vi "Motion Virtual Front Panel_libESP301.vi"() -> ()   [LabVIEW 2015, in "Newport ESP301.lvlib"]
doc: "Motion Virtual Front Panel:\n\nThis is a sample of an application that can be built with the LabVIEW drivers.\n\nPress HOME / ENABLE in top left of panel to put stage in Ready state for motion."
uses:
  <userlib>/Newport ESP301/Newport ESP301.lvlib
  <vilib>/Platform/TimedLoop/XDataNode/timing_clust.ctl
  <vilib>/Platform/TimedLoop/XDataNode/nitl_modes.ctl
  <vilib>/Platform/TimedLoop/XDataNode/wakeup.ctl
  <vilib>/Platform/TimedLoop/XDataNode/XDataNode.xnode
  <vilib>/Platform/TimedLoop/XDataNode/XDNodeRunTimeDep.lvlib
panel:
  out "Title":string
  out "counter":i32
  in  "Set Max":bool
  in  "Set Min":bool
  in  "Max":dbl
  in  "Min":dbl
  in  "Set velocity":bool
  out "Stop cycle":bool=TRUE
  out "Title 2":string
  in  "Cycle":bool
  in  "# Loops":i32=5
  in  "Go2":bool
  in  "Go1":bool
  in  "Abs. Move 2":dbl=1.0
  in  "Abs. Move 1":dbl
  in  "-":bool
  in  "+":bool
  in  "Step":dbl
  out "Position History":dbl(graph)=1.5
  in  "Action":bool
  out "Stop polling":bool=TRUE
  out "Controller state description":string="STATUS"
  out "Velocity MAX":dbl=0.4
  out "Controller state":string="33"
  out "Positioner error":string="0000"
  in  "Velocity:":dbl
  in  "Exit":bool=TRUE
  out "Target position":dbl
  in  "Position glissière":cluster{dbl, dbl}(slide) scale=-45.0..45.0
  in  "Exit":bool
  out "Current position":dbl
  # "unit/s"
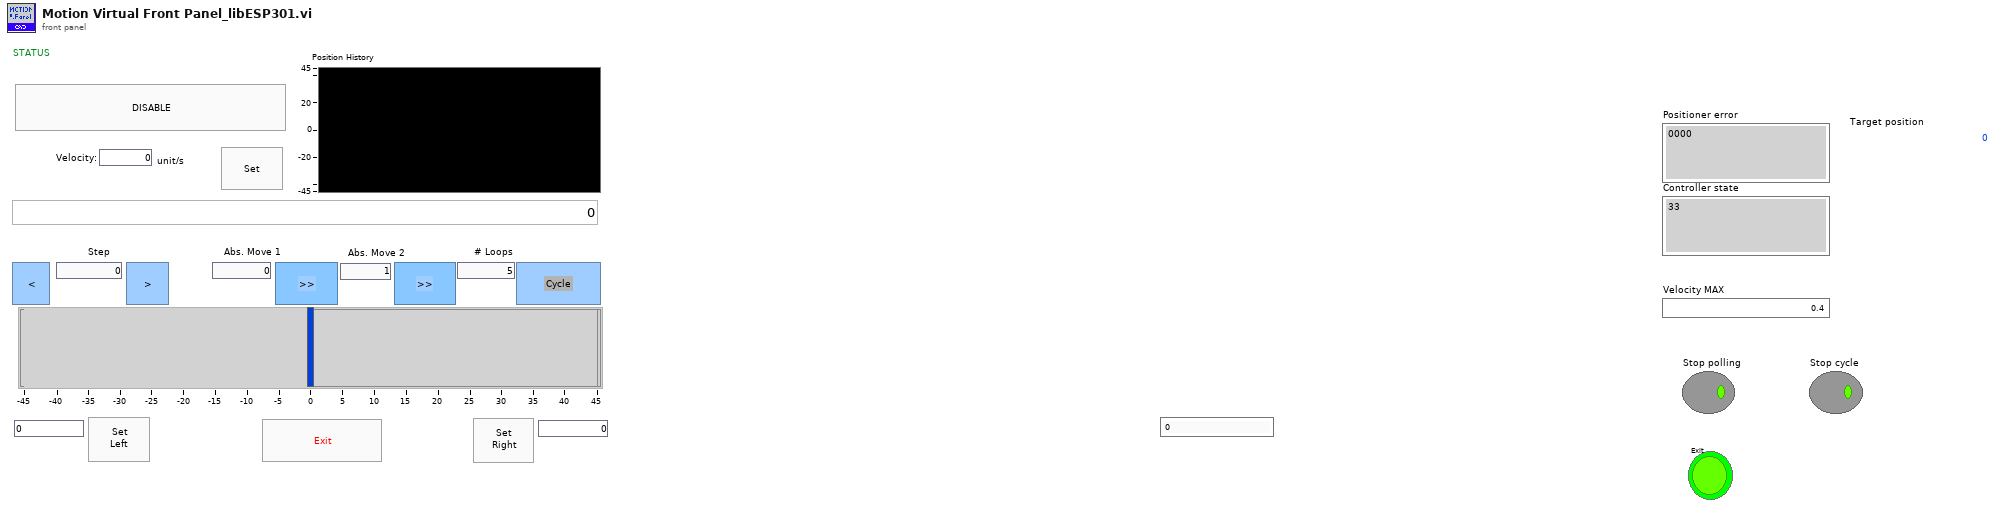
[diagram p1: front panel]
types:
  T1 = typedef "XDNodeRunTimeDep.lvlib/timing_clust.ctl" = cluster{"Expected End [f-1]":u64, "Actual End [f-1]":u64, "Finished Late? [f-1]":bool, "Expected End [i-1]":u64, "Actual End [i-1]":u64, "Finished Late? [i-1]":bool, "Expected Start [i]":u64, "Actual Start [i]":u64, "Expected Start [f]":u64, "Actual Start [f]":u64, "Source Name":string, "Structure Name":string, "Period":i64, "Deadline":i64, "Offset":i64, "Start":i64, "Priority":i32, "Timeout":i32, "Mode":T2, "Wakeup Reason":T3, "Error":errorcluster, "Source Type":string, "Secondary Source Type":string, "Global End Time":u64, "Global Start Time":u64, "Frame Duration":u64, "Iteration Duration":u64, "Assigned CPU":i32, "I/O Scan Engine Mode":u32}
  T2 = typedef "XDNodeRunTimeDep.lvlib/nitl_modes.ctl" = enum32{"No Change", "Process missed periods, maintain original phase", "Discard missed periods, maintain original phase", "Process missed periods, ignore original phase", "Discard missed periods, ignore original phase"}
  T3 = typedef "XDNodeRunTimeDep.lvlib/wakeup.ctl" = enum32{"Normal", "Aborted", "Asynchronous wakeup", "Timing source error", "Timed loop error", "Timeout"}
  T4 = cluster{"VISA resource name":refnum<visa-resource-name>, "Device name":string, "Controller address":i32, "error":errorcluster}
  T5 = cluster{"Axis1 moving":bool, "Axis2 moving":bool, "Axis3 moving":bool, "Axis4 moving":bool, "Motor Power of at least one axis":bool, "Reserved":bool, "Reserved":bool, "Reserved":bool, "Axis5 moving 2":bool, "Axis6 moving 2":bool, "Reserved":bool, "Reserved":bool, "Motor Power of at least one axis":bool, "Reserved":bool, "Reserved":bool, "Reserved":bool}
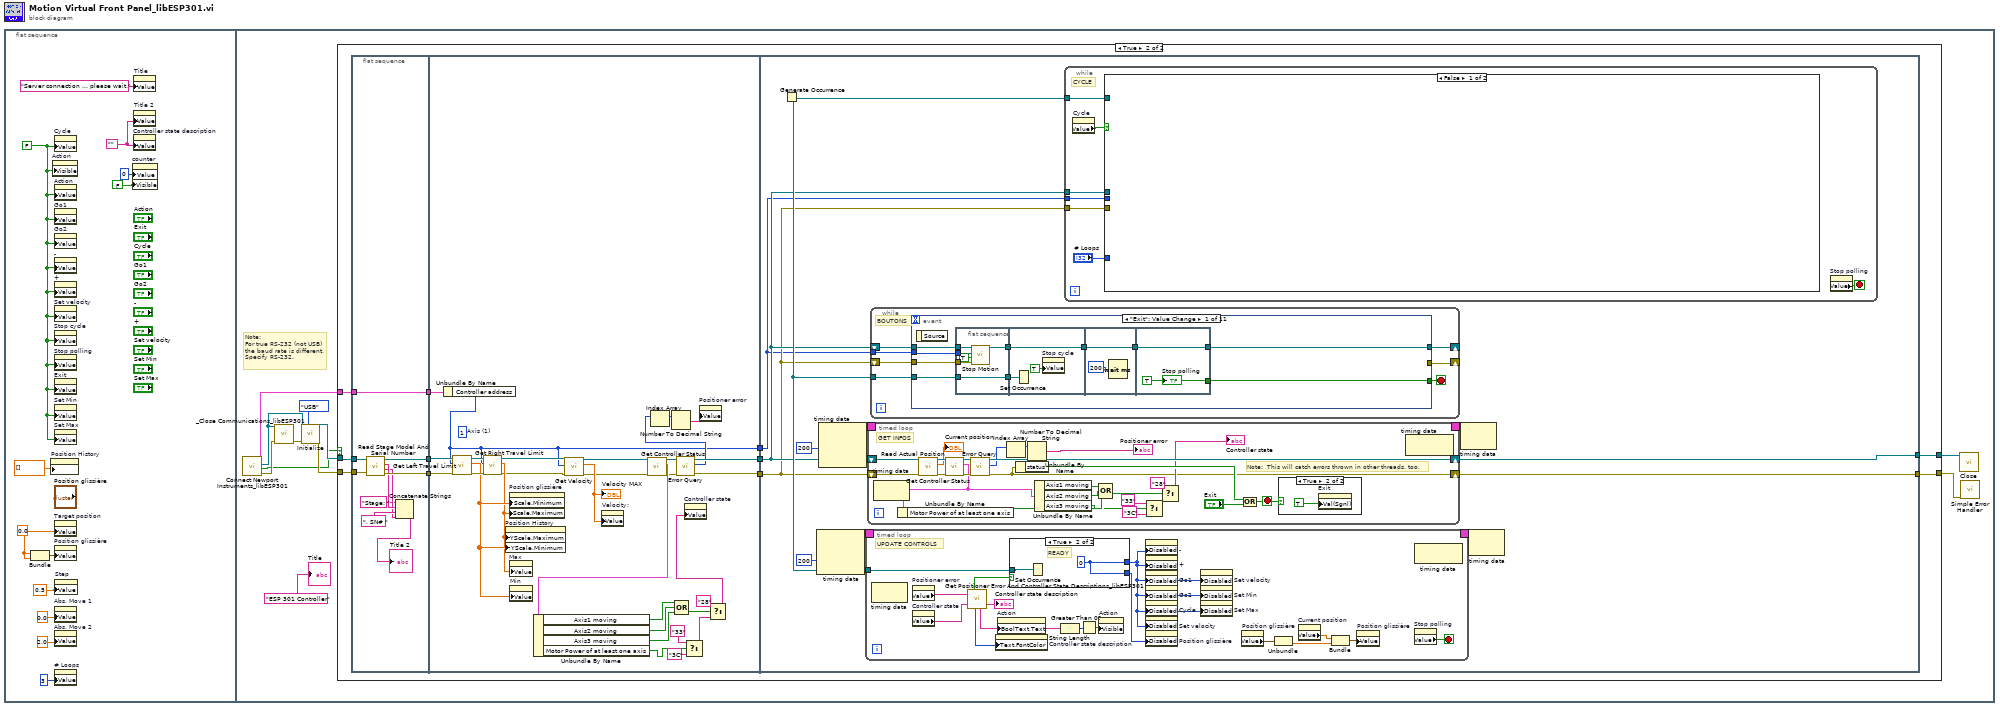
[diagram p0: block diagram]
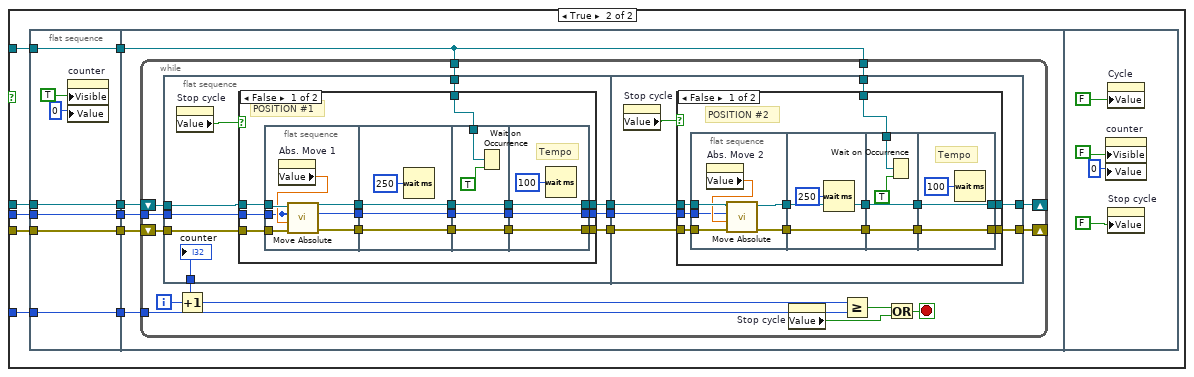
[diagram p3: hidden frame]
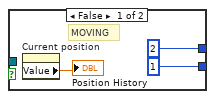
[diagram p6: hidden frame]
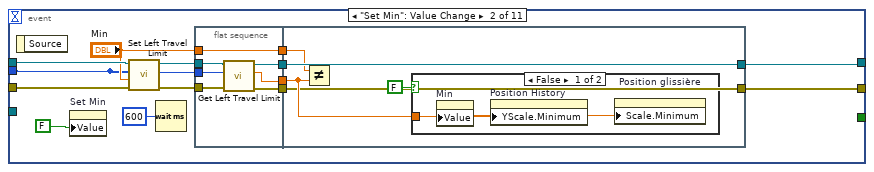
[diagram p7: hidden frame]
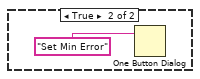
[diagram p8: hidden frame]
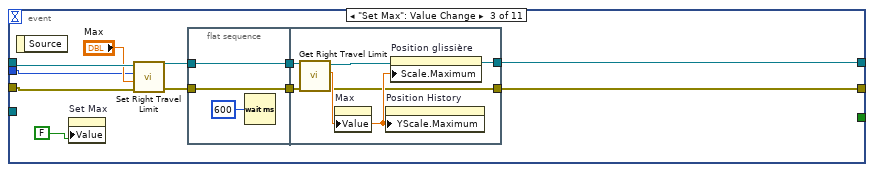
[diagram p9: hidden frame]
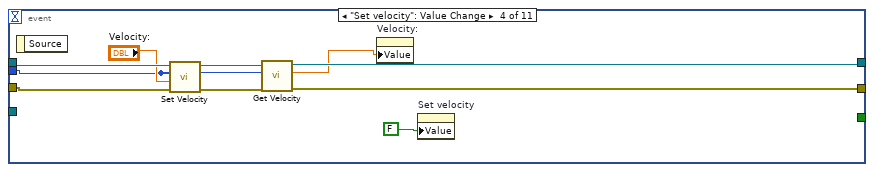
[diagram p10: hidden frame]
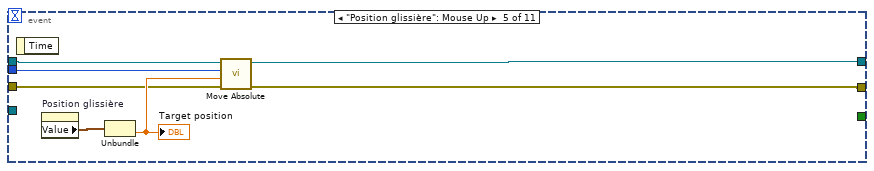
[diagram p11: hidden frame]
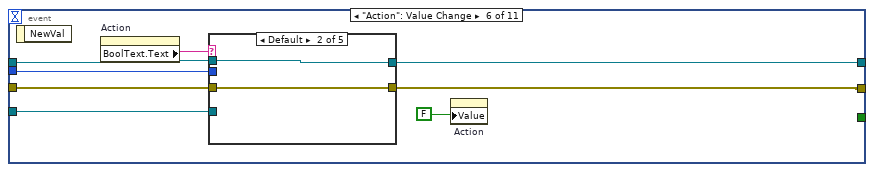
[diagram p12: hidden frame]
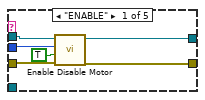
[diagram p13: hidden frame]
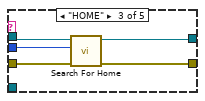
[diagram p14: hidden frame]
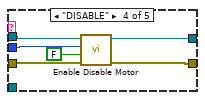
[diagram p15: hidden frame]
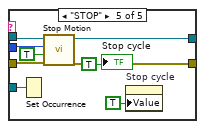
[diagram p16: hidden frame]
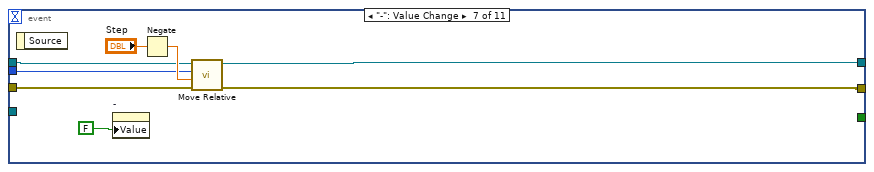
[diagram p17: hidden frame]
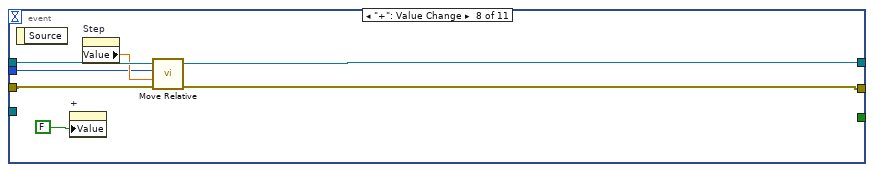
[diagram p18: hidden frame]
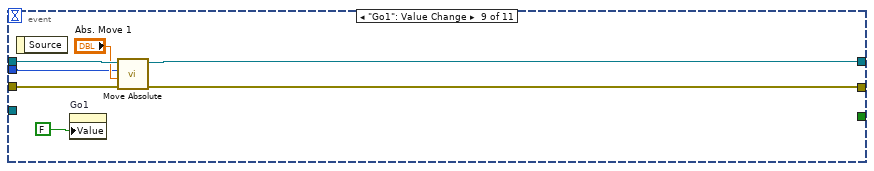
[diagram p19: hidden frame]
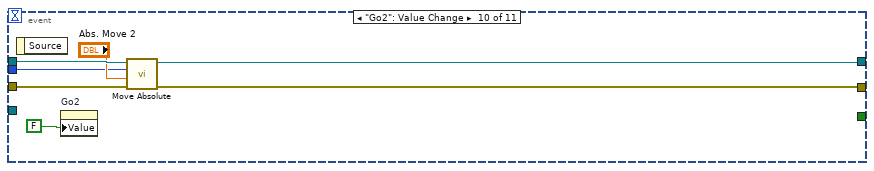
[diagram p20: hidden frame]
diagram:
  n1 = flat-sequence {
    frame #0 {
      w8 = FALSE
      w11 = 0.0
      w10 = ""
      n2 = Bundle(w11, w11) -> (w12:cluster{dbl, dbl})  [unwired: 1 out]
      n3 = property on="Position History" class="WFChart (strict)"("History Data"=dbl[] [] ("Données d'historique")) -> ()  [unwired: 2 in, 2 out]
      n4 = property on="Action" class="Bool (strict)"("Visible"=w8) -> ()  [unwired: 2 in, 2 out]
      n5 = property on="Cycle" class="Bool (strict)"("Value"=w8) -> ()  [unwired: 2 in, 2 out]
      n6 = property on="Action" class="Bool (strict)"("Value"=w8) -> ()  [unwired: 2 in, 2 out]
      n7 = property on="Go1" class="Bool (strict)"("Value"=w8) -> ()  [unwired: 2 in, 2 out]
      n8 = property on="Go2" class="Bool (strict)"("Value"=w8) -> ()  [unwired: 2 in, 2 out]
      n9 = property on="-" class="Bool (strict)"("Value"=w8) -> ()  [unwired: 2 in, 2 out]
      n10 = property on="+" class="Bool (strict)"("Value"=w8) -> ()  [unwired: 2 in, 2 out]
      n11 = property on="Set velocity" class="Bool (strict)"("Value"=w8) -> ()  [unwired: 2 in, 2 out]
      n12 = property on="Stop cycle" class="Bool (strict)"("Value"=w8) -> ()  [unwired: 2 in, 2 out]
      n13 = property on="Stop polling" class="Bool (strict)"("Value"=w8) -> ()  [unwired: 2 in, 2 out]
      n14 = property on="Exit" class="Bool (strict)"("Value"=w8) -> ()  [unwired: 2 in, 2 out]
      n15 = property on="Set Min" class="Bool (strict)"("Value"=w8) -> ()  [unwired: 2 in, 2 out]
      n16 = property on="Set Max" class="Bool (strict)"("Value"=w8) -> ()  [unwired: 2 in, 2 out]
      n17 = property on="Target position" class="DigNum (strict)"("Value"=w11) -> ()  [unwired: 2 in, 2 out]
      n18 = property on="Position glissière" class="Slide (strict)"("Value"=w12) -> ()  [unwired: 2 in, 2 out]
      n19 = property on="Abs. Move 1" class="DigNum (strict)"("Value"=0.0 ("Abs. Move 1")) -> ()  [unwired: 2 in, 2 out]
      n20 = property on="Abs. Move 2" class="DigNum (strict)"("Value"=2.0 ("Abs. Move 2")) -> ()  [unwired: 2 in, 2 out]
      n21 = property on="# Loops" class="DigNum (strict)"("Value"=3 ("# Loops")) -> ()  [unwired: 2 in, 2 out]
      n22 = property on="Step" class="DigNum (strict)"("Value"=0.5 ("Step")) -> ()  [unwired: 2 in, 2 out]
      n23 = property on="counter" class="DigNum (strict)"("Value"=0 ("counter"), "Visible"=FALSE) -> ()  [unwired: 2 in, 2 out]
      n24 = property on="Title" class="Str"("Value"="Server connection ... please wait." ("Title")) -> ()  [unwired: 2 in, 2 out]
      n25 = property on="Title 2" class="Str"("Value"=w10) -> ()  [unwired: 2 in, 2 out]
      n26 = property on="Controller state description" class="Str"("Value"=w10) -> ()  [unwired: 2 in, 2 out]
    }
    frame #1 {
      # "Note:\nFor true RS-232 (not USB)\nthe baud rate is different.\nSpecify RS-232."
      n27 = call <userlib>:"Connect Newport Instruments_libESP301.vi"() -> ("error (duplicate)"=w16:errorcluster, "Connected"=w15:bool, "VISA resource name (duplicate)"=w14:refnum<visa-resource-name>, "Device Connection Cluster"=w13:T4)  [unwired: 7 in, 1 out]
      n28 = call <userlib>:"_Close Communications_libESP301.vi"("Instrument Channel"=w14, "error in (no error)"=w16) -> ("error out"=w22:errorcluster)  [unwired: 13 in]
      n29 = call <userlib>:"Initialize.vi"("VISA resource name"=w14, "error in (no error)"=w22, "Serial Link (USB)"=enum16{"RS232", "USB"}."USB" ("Serial Link (RS232)")) -> ("VISA resource name out"=w20:refnum<visa-resource-name>, "error out"=w19:errorcluster)  [unwired: 6 in]
      n30 = case shown="True" w15 {
        tunnel: w20 -> [w25 w35]
        tunnel: [w25 w33] -> w23
        tunnel: w19 -> [w24 w32]
        tunnel: [w24 w28] -> w18
        tunnel: w13 -> [_ w27]
        frame False {
        }
        frame True {
          n31 = flat-sequence {
            tunnel: w35 -> [w46]
            tunnel: [w45] -> w34
            tunnel: w32 -> [w44]
            tunnel: [w43] -> w31
            tunnel: w27 -> [w37]
            tunnel: [w37] -> w26
            tunnel: [w66] -> w36
            tunnel: w34 -> [w77]
            tunnel: w31 -> [w75]
            tunnel: [w49] -> w30
            tunnel: [w47] -> w29
            tunnel: w26 -> [w48]
            tunnel: [w89] -> w33
            tunnel: [w88] -> w28
            tunnel: w29 -> [w78]
            tunnel: w30 -> [w79]
            tunnel: w36 -> [w80]
            frame #0 {
              n32 = call <userlib>:"Read Stage Model And Serial Number.vi"("error in (no error)"=w44, "VISA resource name"=w46) -> ("error out"=w43:errorcluster, "Serial number"=w40:string, "Model number"=w41:string, "VISA resource name out"=w45:refnum<visa-resource-name>)  [unwired: 2 in]
              n33 = Concatenate Strings("Stage: " ("string"), w41, ", SN# " ("string"), w40) -> (→"Title 2":string)
            }
            frame #1 {
              (unwired) 1  # Axis (1)
              n34 = Unbundle By Name(w48) -> ("Controller address"=w47:i32)
              n35 = call <userlib>:"Get Left Travel Limit.vi"("error in (no error)"=w75, "Axis (1)"=w47, "VISA resource name"=w77) -> ("error out"=w74:errorcluster, "Left Travel Limit (units)"=w73:dbl, "VISA resource name out"=w76:refnum<visa-resource-name>)  [unwired: 2 in]
              n36 = call <userlib>:"Get Right Travel Limit.vi"("error in (no error)"=w74, "Axis (1)"=w47, "VISA resource name"=w76) -> ("error out"=w68:errorcluster, "Right Travel Limit (units)"=w72:dbl, "VISA resource name out"=w71:refnum<visa-resource-name>)  [unwired: 2 in]
              n37 = property on="Position History" class="WFChart (strict)"("YScale.Maximum"=w72, "YScale.Minimum"=w73) -> ()  [unwired: 2 in, 2 out]
              n38 = property on="Position glissière" class="Slide (strict)"("Scale.Minimum"=w73, "Scale.Maximum"=w72) -> ()  [unwired: 2 in, 2 out]
              n39 = property on="Max" class="DigNum (strict)"("Value"=w72) -> ()  [unwired: 2 in, 2 out]
              n40 = property on="Min" class="DigNum (strict)"("Value"=w73) -> ()  [unwired: 2 in, 2 out]
              n41 = call <userlib>:"Get Velocity.vi"("error in (no error)"=w68, "Axis (1)"=w47, "VISA resource name"=w71) -> ("error out"=w51:errorcluster, "Velocity (units/s)"=w69:dbl, "VISA resource name out"=w70:refnum<visa-resource-name>)  [unwired: 2 in]
              "Velocity MAX" <- w69
              n42 = property on="Velocity:" class="DigNum (strict)"("Value"=w69) -> ()  [unwired: 2 in, 2 out]
              n43 = call <userlib>:"Get Controller Status.vi"("error in (no error)"=w51, "VISA resource name"=w70) -> ("error out"=w50:errorcluster, "Controller Status"=w62:T5, "VISA resource name out"=w67:refnum<visa-resource-name>)  [unwired: 2 in, 1 out]
              n44 = Unbundle By Name(w62) -> ("Axis1 moving"=w61:bool, "Axis2 moving"=w60:bool, "Axis3 moving"=w59:bool, "Motor Power of at least one axis"=w52:bool)
              n45 = Compound Arithmetic op=OR(w61, w60, w59) -> (w58:bool)
              n46 = call <userlib>:"Error Query.vi"("error in (no error)"=w50, "VISA resource name"=w67) -> ("error out"=w49:errorcluster, "Error Code"=w64:i32[], "VISA resource name out"=w66:refnum<visa-resource-name>)  [unwired: 2 in, 1 out]
              n47 = Index Array(array=w64) -> (element=w65:i32)  [unwired: 1 in]
              n48 = Number To Decimal String(number=w65) -> (decimal integer string=w63:string)  [unwired: 1 in]
              n49 = Select(t="33" ("f"), s=w52, f="3C") -> (s? t:f=w54:string)
              n50 = property on="Positioner error" class="Str"("Value"=w63) -> ()  [unwired: 2 in, 2 out]
              n51 = Select(t="28", s=w58, f=w54) -> (s? t:f=w56:string)
              n52 = property on="Controller state" class="Str"("Value"=w56) -> ()  [unwired: 2 in, 2 out]
            }
            frame #2 {
              n53 = Generate Occurrence() -> (w81:refnum<k4>)
              n54 = node-c288(i64 200 ("Période")) -> (w85:T1)  [unwired: 1 in, 1 out]
              n55 = node-c288(i64 200 ("Période")) -> (w87:T1)  [unwired: 1 in, 1 out]
              n56 = timed-loop {
                timing: w85 -> [_]
                timing-out: [_] -> w84
                tunnel: w81 -> [w227]
                stop <- w229 stop-if-true
                # "UPDATE CONTROLS"
                n57 = node-c288() -> ()  [unwired: 2 out]
                n58 = property on="Positioner error" class="Str"() -> ("Value"=w238:string)  [unwired: 2 in, 2 out]
                n59 = property on="Controller state" class="Str"() -> ("Value"=w237:string)  [unwired: 2 in, 2 out]
                n60 = call <userlib>:"Get Positioner Error And Controller State Descriptions_libESP301.vi"("Controller state"=w237, "Positioner error"=w238) -> ("Color"=w235:u32, "Action name"=w234:string, "Controller state description"=→"Controller state description":string, "IsReady?"=w231:bool)  [unwired: 2 out]
                n61 = property on="Controller state description" class="Str"("Text.FontColor"=w235) -> ()  [unwired: 2 in, 2 out]
                n62 = property on="Action" class="Bool (strict)"("BoolText.Text"=w234) -> ()  [unwired: 2 in, 2 out]
                n63 = case shown="True" w231 {
                  tunnel: [u8 2 w243] -> w228
                  tunnel: [u8 1 w243] -> w230
                  tunnel: w227 -> [_ w242]
                  frame False {
                    # "MOVING"
                    n64 = property on="Current position" class="DigNum (strict)"() -> ("Value"=→"Position History":dbl)  [unwired: 2 in, 2 out]
                  }
                  frame True {
                    w243 = u8 0
                    # "READY"
                    n65 = Set Occurrence(w242) -> ()
                  }
                }
                n66 = String Length(string=w234) -> (length=w233:i32)
                n67 = Greater Than 0?(x=w233) -> (x > 0?=w232:bool)
                n68 = property on="Action" class="Bool (strict)"("Visible"=w232) -> ()  [unwired: 2 in, 2 out]
                n69 = property on="-" class="Bool (strict)"("Disabled"=w228) -> ()  [unwired: 2 in, 2 out]
                n70 = property on="+" class="Bool (strict)"("Disabled"=w228) -> ()  [unwired: 2 in, 2 out]
                n71 = property on="Go1" class="Bool (strict)"("Disabled"=w228) -> ()  [unwired: 2 in, 2 out]
                n72 = property on="Go2" class="Bool (strict)"("Disabled"=w228) -> ()  [unwired: 2 in, 2 out]
                n73 = property on="Cycle" class="Bool (strict)"("Disabled"=w228) -> ()  [unwired: 2 in, 2 out]
                n74 = property on="Set velocity" class="Bool (strict)"("Disabled"=w228) -> ()  [unwired: 2 in, 2 out]
                n75 = property on="Position glissière" class="Slide (strict)"("Disabled"=w230) -> ()  [unwired: 2 in, 2 out]
                n76 = property on="Set velocity" class="Bool (strict)"("Disabled"=w228) -> ()  [unwired: 2 in, 2 out]
                n77 = property on="Set Min" class="Bool (strict)"("Disabled"=w228) -> ()  [unwired: 2 in, 2 out]
                n78 = property on="Set Max" class="Bool (strict)"("Disabled"=w228) -> ()  [unwired: 2 in, 2 out]
                n79 = property on="Position glissière" class="Slide (strict)"() -> ("Value"=w224:cluster{dbl, dbl})  [unwired: 2 in, 2 out]
                n80 = Unbundle(w224) -> (w223:dbl)  [unwired: 1 out]
                n81 = property on="Current position" class="DigNum (strict)"() -> ("Value"=w225:dbl)  [unwired: 2 in, 2 out]
                n82 = Bundle("Value"=w225, w223) -> (w226:cluster{"Value":dbl, dbl})  [unwired: 1 out]
                n83 = property on="Position glissière" class="Slide (strict)"("Value"=w226) -> ()  [unwired: 2 in, 2 out]
                n84 = node-c288() -> ()  [unwired: 2 out]
                n85 = property on="Stop polling" class="Bool (strict)"() -> ("Value"=w229:bool)  [unwired: 2 in, 2 out]
              }
              n86 = timed-loop {
                timing: w87 -> [_]
                timing-out: [_] -> w86
                shift-right: [w427] -> w89
                shift-left: w80 -> [w434]
                shift-right: [w411] -> w88
                shift-left: w79 -> [w412]
                stop <- w436 stop-if-true
                # "Note:  This will catch errors thrown in other threads, too."
                # "GET INFOS"
                n87 = node-c288() -> ()  [unwired: 2 out]
                n88 = call <userlib>:"Read Actual Position.vi"("error in (no error)"=w412, "VISA resource name"=w434) -> ("error out"=w431:errorcluster, "Position (units)"=→"Current position":dbl, "VISA resource name out"=w433:refnum<visa-resource-name>)  [unwired: 3 in]
                n89 = call <userlib>:"Get Controller Status.vi"("error in (no error)"=w431, "VISA resource name"=w433) -> ("error out"=w428:errorcluster, "Controller Status"=w417:T5, "VISA resource name out"=w429:refnum<visa-resource-name>)  [unwired: 2 in, 1 out]
                n90 = Unbundle By Name(w417) -> ("Motor Power of at least one axis"=w416:bool)
                n91 = call <userlib>:"Error Query.vi"("error in (no error)"=w428, "VISA resource name"=w429) -> ("error out"=w411:errorcluster, "Error Code"=w426:i32[], "VISA resource name out"=w427:refnum<visa-resource-name>)  [unwired: 2 in, 1 out]
                n92 = Index Array(array=w426) -> (element=w425:i32)  [unwired: 1 in]
                n93 = Unbundle By Name(w411) -> ("status"=w430:bool)
                n94 = Number To Decimal String(number=w425) -> (decimal integer string=→"Positioner error":string)  [unwired: 1 in]
                n95 = Unbundle By Name(w417) -> ("Axis1 moving"=w419:bool, "Axis2 moving"=w420:bool, "Axis3 moving"=w421:bool)
                n96 = Compound Arithmetic op=OR(w419, w420, w421) -> (w422:bool)
                n97 = Select(t="33" ("f"), s=w416, f="3C") -> (s? t:f=w413:string)
                n98 = Select(t="28", s=w422, f=w413) -> (s? t:f=→"Controller state":string)
                n99 = Or(x=w430, y="Exit") -> (x .or. y?=w436:bool)
                n100 = case shown="True" w436 {
                  frame False {
                  }
                  frame True {
                    n101 = property on="Exit" class="Bool (strict)"("Val(Sgnl)"=TRUE) -> ()  [unwired: 2 in, 2 out]
                  }
                }
                n102 = node-c288() -> ()  [unwired: 2 out]
              }
              n103 = while {
                shift-right: [w256] -> _
                shift-left: w80 -> [w255]
                tunnel: w81 -> [w253]
                tunnel: w78 -> [w251]
                shift-right: [w250] -> _
                shift-left: w79 -> [w252]
                stop <- w254 stop-if-true
                # "BOUTONS"
                n104 = event shown="[0] \"Exit\": Value Change" {
                  selector: _ -> [_ _ _ _ _ _ _ _ _ _ _]
                  dyn-events: _ -> [_ _ _ _ _ _ _ _ _ _ _]
                  timeout: _ -> [_ _ _ _ _ _ _ _ _ _ _]
                  tunnel: [w264 _ _ _ _ _ _ _ _ _ _] -> w254
                  tunnel: w255 -> [w259 w287 w315 w335 w342 w350 w384 w392 w400 w406 w409]
                  tunnel: [w266 w292 w316 w333 w341 w349 w383 w393 w399 w407 w409] -> w256
                  tunnel: w253 -> [w261 _ _ _ _ w347 _ _ _ _ _]
                  tunnel: w252 -> [w257 w283 w312 w330 w338 w346 w382 w390 w397 w404 _]
                  tunnel: w251 -> [w258 w284 w311 w327 w339 w345 w381 w389 w395 w403 _]
                  tunnel: [_ w281 w308 w328 w337 w344 w380 w388 w396 w402 _] -> w250
                  event "Exit": Value Change {
                    n105 = event-data() -> ()  [unwired: 2 out]
                    n106 = flat-sequence {
                      tunnel: [w270] -> w265
                      tunnel: w261 -> [w272]
                      tunnel: [w272] -> w260
                      tunnel: w259 -> [w271]
                      tunnel: w258 -> [w268]
                      tunnel: w257 -> [w267]
                      tunnel: w265 -> [w275]
                      tunnel: [w275] -> w263
                      tunnel: w260 -> [w273]
                      tunnel: w263 -> [w277]
                      tunnel: [w277] -> w262
                      tunnel: [w279] -> w266
                      tunnel: w262 -> [w279]
                      tunnel: [w278] -> w264
                      frame #0 {
                        n107 = call <userlib>:"Stop Motion.vi"("error in (no error)"=w267, "Stop all axes (F)"=TRUE, "Axis (1)"=w268, "VISA resource name"=w271) -> ("VISA resource name out"=w270:refnum<visa-resource-name>)  [unwired: 2 in, 1 out]
                      }
                      frame #1 {
                        n108 = Set Occurrence(w273) -> ()
                        n109 = property on="Stop cycle" class="Bool (strict)"("Value"=TRUE) -> ()  [unwired: 2 in, 2 out]
                      }
                      frame #2 {
                        n110 = Wait (ms)(milliseconds to wait=u32 200 ("attente (ms)")) -> ()  [unwired: 1 out]
                      }
                      frame #3 {
                        w278 = TRUE
                        "Stop polling" <- w278
                      }
                    }
                  }
                  event "Set Min": Value Change {
                    n111 = event-data() -> ()  [unwired: 2 out]
                    n112 = property on="Set Min" class="Bool (strict)"("Value"=FALSE ("Set Min")) -> ()  [unwired: 2 in, 2 out]
                    n113 = call <userlib>:"Set Left Travel Limit.vi"("error in (no error)"=w283, "Left Travel Limit"="Min", "Axis (1)"=w284, "VISA resource name"=w287) -> ("error out"=w282:errorcluster, "VISA resource name out"=w286:refnum<visa-resource-name>)  [unwired: 2 in]
                    n114 = Wait (ms)(milliseconds to wait=u32 600 ("attente (ms)")) -> ()  [unwired: 1 out]
                    n115 = flat-sequence {
                      tunnel: [w298] -> w290
                      tunnel: [w300] -> w289
                      tunnel: "Min" -> [w300]
                      tunnel: [w297] -> w288
                      tunnel: w286 -> [w299]
                      tunnel: w284 -> [w296]
                      tunnel: w282 -> [w295]
                      tunnel: [w294] -> w280
                      tunnel: [w305] -> w292
                      tunnel: w290 -> [w305]
                      tunnel: w289 -> [w304]
                      tunnel: w288 -> [w302]
                      tunnel: [w301] -> w281
                      tunnel: w280 -> [w301]
                      frame #0 {
                        n116 = call <userlib>:"Get Left Travel Limit.vi"("error in (no error)"=w295, "Axis (1)"=w296, "VISA resource name"=w299) -> ("error out"=w294:errorcluster, "Left Travel Limit (units)"=w297:dbl, "VISA resource name out"=w298:refnum<visa-resource-name>)  [unwired: 2 in]
                      }
                      frame #1 {
                        n117 = Not Equal?(x=w304, y=w302) -> ()  [unwired: 1 out]
                        n118 = case shown="False" FALSE {
                          tunnel: w302 -> [w306 _]
                          frame False {
                            n119 = property on="Min" class="DigNum (strict)"("Value"=w306) -> ()  [unwired: 2 in, 2 out]
                            n120 = property on="Position History" class="WFChart (strict)"("YScale.Minimum"=w306) -> ()  [unwired: 2 in, 2 out]
                            n121 = property on="Position glissière" class="Slide (strict)"("Scale.Minimum"=w306) -> ()  [unwired: 2 in, 2 out]
                          }
                          frame True {
                            n122 = One Button Dialog(message="Set Min Error") -> ()  [unwired: 1 in, 1 out]
                          }
                        }
                      }
                    }
                  }
                  event "Set Max": Value Change {
                    n123 = event-data() -> ()  [unwired: 2 out]
                    n124 = property on="Set Max" class="Bool (strict)"("Value"=FALSE ("Set Max")) -> ()  [unwired: 2 in, 2 out]
                    n125 = call <userlib>:"Set Right Travel Limit.vi"("error in (no error)"=w312, "Right Travel Limit"="Max", "Axis (1)"=w311, "VISA resource name"=w315) -> ("error out"=w310:errorcluster, "VISA resource name out"=w314:refnum<visa-resource-name>)  [unwired: 2 in]
                    n126 = flat-sequence {
                      tunnel: w314 -> [w321]
                      tunnel: [w321] -> w317
                      tunnel: w310 -> [w319]
                      tunnel: [w319] -> w309
                      tunnel: [w325] -> w316
                      tunnel: w317 -> [w326]
                      tunnel: w309 -> [w323]
                      tunnel: [w322] -> w308
                      frame #0 {
                        n127 = Wait (ms)(milliseconds to wait=u32 600 ("attente (ms)")) -> ()  [unwired: 1 out]
                      }
                      frame #1 {
                        n128 = call <userlib>:"Get Right Travel Limit.vi"("error in (no error)"=w323, "VISA resource name"=w326) -> ("error out"=w322:errorcluster, "Right Travel Limit (units)"=w324:dbl, "VISA resource name out"=w325:refnum<visa-resource-name>)  [unwired: 3 in]
                        n129 = property on="Max" class="DigNum (strict)"("Value"=w324) -> ()  [unwired: 2 in, 2 out]
                        n130 = property on="Position History" class="WFChart (strict)"("YScale.Maximum"=w324) -> ()  [unwired: 2 in, 2 out]
                        n131 = property on="Position glissière" class="Slide (strict)"("Scale.Maximum"=w324) -> ()  [unwired: 2 in, 2 out]
                      }
                    }
                  }
                  event "Set velocity": Value Change {
                    n132 = event-data() -> ()  [unwired: 2 out]
                    n133 = call <userlib>:"Set Velocity.vi"("error in (no error)"=w330, "Velocity (units/s)"="Velocity:", "Axis (1)"=w327, "VISA resource name"=w335) -> ("error out"=w329:errorcluster, "VISA resource name out"=w334:refnum<visa-resource-name>)  [unwired: 2 in]
                    n134 = call <userlib>:"Get Velocity.vi"("error in (no error)"=w329, "Axis (1)"=w327, "VISA resource name"=w334) -> ("error out"=w328:errorcluster, "Velocity (units/s)"=w331:dbl, "VISA resource name out"=w333:refnum<visa-resource-name>)  [unwired: 2 in]
                    n135 = property on="Velocity:" class="DigNum (strict)"("Value"=w331) -> ()  [unwired: 2 in, 2 out]
                    n136 = property on="Set velocity" class="Bool (strict)"("Value"=FALSE ("Set velocity")) -> ()  [unwired: 2 in, 2 out]
                  }
                  event "Position glissière": Mouse Up {
                    n137 = event-data() -> ()  [unwired: 2 out]
                    n138 = property on="Position glissière" class="Slide (strict)"() -> ("Value"=w343:cluster{dbl, dbl})  [unwired: 2 in, 2 out]
                    n139 = Unbundle(w343) -> (w340:dbl)  [unwired: 1 out]
                    "Target position" <- w340
                    n140 = call <userlib>:"Move Absolute.vi"("error in (no error)"=w338, "Position (0 units)"=w340, "Axis (1)"=w339, "VISA resource name"=w342) -> ("error out"=w337:errorcluster, "VISA resource name out"=w341:refnum<visa-resource-name>)  [unwired: 2 in]
                  }
                  event "Action": Value Change {
                    n141 = event-data() -> ()  [unwired: 2 out]
                    n142 = property on="Action" class="Bool (strict)"() -> ("BoolText.Text"=w351:string)  [unwired: 2 in, 2 out]
                    n143 = case shown="Default" w351 {
                      tunnel: w350 -> [w357 w359 w364 w370 w376]
                      tunnel: [w356 w359 w363 w369 w375] -> w349
                      tunnel: w347 -> [_ _ _ _ w378]
                      tunnel: w346 -> [w353 w358 w362 w367 w372]
                      tunnel: w345 -> [w352 _ w361 w366 w371]
                      tunnel: [w354 w358 w360 w365 w373] -> w344
                      frame "ENABLE" {
                        n144 = call <userlib>:"Enable Disable Motor.vi"("error in (no error)"=w353, "Action (F - OFF)"=TRUE ("Flag (false=DISABLE true=READY)"), "Axis (1)"=w352, "VISA resource name"=w357) -> ("error out"=w354:errorcluster, "VISA resource name out"=w356:refnum<visa-resource-name>)  [unwired: 2 in]
                      }
                      frame Default {
                      }
                      frame "HOME" {
                        n145 = call <userlib>:"Search For Home.vi"("error in (no error)"=w362, "Axis (1)"=w361, "VISA resource name"=w364) -> ("error out"=w360:errorcluster, "VISA resource name out"=w363:refnum<visa-resource-name>)  [unwired: 4 in]
                      }
                      frame "DISABLE" {
                        n146 = call <userlib>:"Enable Disable Motor.vi"("error in (no error)"=w367, "Action (F - OFF)"=FALSE ("Flag (false=DISABLE true=READY)"), "Axis (1)"=w366, "VISA resource name"=w370) -> ("error out"=w365:errorcluster, "VISA resource name out"=w369:refnum<visa-resource-name>)  [unwired: 2 in]
                      }
                      frame "STOP" {
                        n147 = Set Occurrence(w378) -> ()
                        n148 = call <userlib>:"Stop Motion.vi"("error in (no error)"=w372, "Stop all axes (F)"=TRUE, "Axis (1)"=w371, "VISA resource name"=w376) -> ("error out"=w373:errorcluster, "VISA resource name out"=w375:refnum<visa-resource-name>)  [unwired: 2 in]
                        n149 = property on="Stop cycle" class="Bool (strict)"("Value"=TRUE) -> ()  [unwired: 2 in, 2 out]
                        "Stop cycle" <- TRUE ("Stop cycle")
                      }
                    }
                    n150 = property on="Action" class="Bool (strict)"("Value"=FALSE) -> ()  [unwired: 2 in, 2 out]
                  }
                  event "-": Value Change {
                    n151 = event-data() -> ()  [unwired: 2 out]
                    n152 = property on="-" class="Bool (strict)"("Value"=FALSE ("-")) -> ()  [unwired: 2 in, 2 out]
                    n153 = Negate(x="Step") -> (-x=w385:dbl)
                    n154 = call <userlib>:"Move Relative.vi"("error in (no error)"=w382, "Position (0 units)"=w385, "Axis (1)"=w381, "VISA resource name"=w384) -> ("error out"=w380:errorcluster, "VISA resource name out"=w383:refnum<visa-resource-name>)  [unwired: 2 in]
                  }
                  event "+": Value Change {
                    n155 = event-data() -> ()  [unwired: 2 out]
                    n156 = property on="+" class="Bool (strict)"("Value"=FALSE ("+")) -> ()  [unwired: 2 in, 2 out]
                    n157 = property on="Step" class="DigNum (strict)"() -> ("Value"=w391:dbl)  [unwired: 2 in, 2 out]
                    n158 = call <userlib>:"Move Relative.vi"("error in (no error)"=w390, "Position (0 units)"=w391, "Axis (1)"=w389, "VISA resource name"=w392) -> ("error out"=w388:errorcluster, "VISA resource name out"=w393:refnum<visa-resource-name>)  [unwired: 2 in]
                  }
                  event "Go1": Value Change {
                    n159 = event-data() -> ()  [unwired: 2 out]
                    n160 = property on="Go1" class="Bool (strict)"("Value"=FALSE ("Go1")) -> ()  [unwired: 2 in, 2 out]
                    n161 = call <userlib>:"Move Absolute.vi"("error in (no error)"=w397, "Position (0 units)"="Abs. Move 1", "Axis (1)"=w395, "VISA resource name"=w400) -> ("error out"=w396:errorcluster, "VISA resource name out"=w399:refnum<visa-resource-name>)  [unwired: 2 in]
                  }
                  event "Go2": Value Change {
                    n162 = event-data() -> ()  [unwired: 2 out]
                    n163 = property on="Go2" class="Bool (strict)"("Value"=FALSE ("Go2")) -> ()  [unwired: 2 in, 2 out]
                    n164 = call <userlib>:"Move Absolute.vi"("error in (no error)"=w404, "Position (0 units)"="Abs. Move 2", "Axis (1)"=w403, "VISA resource name"=w406) -> ("error out"=w402:errorcluster, "VISA resource name out"=w407:refnum<visa-resource-name>)  [unwired: 2 in]
                  }
                  event "Cycle": Value Change {
                    n165 = event-data() -> ()  [unwired: 2 out]
                    n166 = property on="Cycle" class="Bool (strict)"("Value"=TRUE ("Cycle")) -> ()  [unwired: 2 in, 2 out]
                  }
                }
              }
              n167 = while {
                tunnel: w80 -> [w96]
                tunnel: w81 -> [w92]
                tunnel: w79 -> [w91]
                tunnel: w78 -> [w90]
                stop <- w95 stop-if-true
                # "CYCLE"
                n168 = property on="Cycle" class="Bool (strict)"() -> ("Value"=w94:bool)  [unwired: 2 in, 2 out]
                n169 = case shown="False" w94 {
                  tunnel: w96 -> [_ w106]
                  tunnel: "# Loops" -> [_ w105]
                  tunnel: w92 -> [_ w102]
                  tunnel: w91 -> [_ w100]
                  tunnel: w90 -> [_ w98]
                  frame False {
                  }
                  frame True {
                    n170 = flat-sequence {
                      tunnel: w105 -> [w112]
                      tunnel: w106 -> [w113]
                      tunnel: [w113] -> w104
                      tunnel: [w112] -> w103
                      tunnel: w102 -> [w109]
                      tunnel: [w109] -> w101
                      tunnel: w100 -> [w108]
                      tunnel: [w108] -> w99
                      tunnel: w98 -> [w107]
                      tunnel: [w107] -> w97
                      tunnel: w104 -> [w116]
                      tunnel: w103 -> [w118]
                      tunnel: w101 -> [w117]
                      tunnel: w99 -> [w115]
                      tunnel: w97 -> [w114]
                      frame #0 {
                        n171 = property on="counter" class="DigNum (strict)"("Visible"=TRUE, "Value"=0 ("counter")) -> ()  [unwired: 2 in, 2 out]
                      }
                      frame #1 {
                        n172 = while {
                          tunnel: w118 -> [w134]
                          shift-right: [w124] -> _
                          shift-left: w116 -> [w125]
                          tunnel: w117 -> [w130]
                          tunnel: w117 -> [w129]
                          tunnel: w114 -> [w122]
                          shift-right: [w119] -> _
                          shift-left: w115 -> [w123]
                          i -> [w128]
                          stop <- w133 stop-if-true
                          n173 = flat-sequence {
                            tunnel: [w143] -> w126
                            tunnel: w130 -> [w141]
                            tunnel: w127 -> [w140]
                            tunnel: w125 -> [w139]
                            tunnel: w123 -> [w138]
                            tunnel: w122 -> [w137]
                            tunnel: [w136] -> w121
                            tunnel: [w135] -> w120
                            tunnel: w126 -> [w188]
                            tunnel: w129 -> [w186]
                            tunnel: [w185] -> w124
                            tunnel: w121 -> [w184]
                            tunnel: w120 -> [w183]
                            tunnel: [w182] -> w119
                            frame #0 {
                              n174 = property on="Stop cycle" class="Bool (strict)"() -> ("Value"=w142:bool)  [unwired: 2 in, 2 out]
                              n175 = case shown="False" w142 {
                                tunnel: w139 -> [w159 w181]
                                tunnel: [w158 w181] -> w143
                                tunnel: w141 -> [w157 _]
                                tunnel: w138 -> [w153 w179]
                                tunnel: w137 -> [w152 w180]
                                tunnel: [w148 w179] -> w136
                                tunnel: [w144 w180] -> w135
                                frame False {
                                # "POSITION #1"
                                n176 = flat-sequence {
                                tunnel: w159 -> [w164]
                                tunnel: [w165] -> w156
                                tunnel: w153 -> [w162]
                                tunnel: w152 -> [w160]
                                tunnel: [w161] -> w151
                                tunnel: [w160] -> w147
                                tunnel: w156 -> [w169]
                                tunnel: [w169] -> w155
                                tunnel: w151 -> [w167]
                                tunnel: [w167] -> w150
                                tunnel: w147 -> [w166]
                                tunnel: [w166] -> w146
                                tunnel: w155 -> [w174]
                                tunnel: w157 -> [w172]
                                tunnel: [w174] -> w154
                                tunnel: w150 -> [w171]
                                tunnel: [w171] -> w149
                                tunnel: w146 -> [w170]
                                tunnel: [w170] -> w145
                                tunnel: [w178] -> w158
                                tunnel: w154 -> [w178]
                                tunnel: w149 -> [w176]
                                tunnel: [w176] -> w148
                                tunnel: w145 -> [w175]
                                tunnel: [w175] -> w144
                                frame #0 {
                                n177 = property on="Abs. Move 1" class="DigNum (strict)"() -> ("Value"=w163:dbl)  [unwired: 2 in, 2 out]
                                n178 = call <userlib>:"Move Absolute.vi"("error in (no error)"=w162, "Position (0 units)"=w163, "Axis (1)"=w160, "VISA resource name"=w164) -> ("error out"=w161:errorcluster, "VISA resource name out"=w165:refnum<visa-resource-name>)  [unwired: 2 in]
                                }
                                frame #1 {
                                n179 = Wait (ms)(milliseconds to wait=u32 250 ("attente (ms)")) -> ()  [unwired: 1 out]
                                }
                                frame #2 {
                                n180 = Wait on Occurrence(1:TRUE ("ignorer les précédents (V)"), 2:w172) -> ()  [unwired: 1 in, 1 out]
                                }
                                frame #3 {
                                # "Tempo"
                                n181 = Wait (ms)(milliseconds to wait=u32 100 ("attente (ms)")) -> ()  [unwired: 1 out]
                                }
                                }
                                }
                                frame True {
                                }
                              }
                              "counter" <- w140
                            }
                            frame #1 {
                              n182 = property on="Stop cycle" class="Bool (strict)"() -> ("Value"=w187:bool)  [unwired: 2 in, 2 out]
                              n183 = case shown="False" w187 {
                                tunnel: w188 -> [w200 w218]
                                tunnel: w186 -> [w199 _]
                                tunnel: [w198 w218] -> w185
                                tunnel: w184 -> [w194 w217]
                                tunnel: w183 -> [w193 _]
                                tunnel: [w192 w217] -> w182
                                frame False {
                                # "POSITION #2"
                                n184 = flat-sequence {
                                tunnel: w200 -> [w206]
                                tunnel: [w205] -> w195
                                tunnel: w194 -> [w203]
                                tunnel: w193 -> [w202]
                                tunnel: [w201] -> w189
                                tunnel: [w208] -> w196
                                tunnel: w195 -> [w208]
                                tunnel: [w207] -> w190
                                tunnel: w189 -> [w207]
                                tunnel: w199 -> [w213]
                                tunnel: [w211] -> w197
                                tunnel: w196 -> [w211]
                                tunnel: [w210] -> w191
                                tunnel: w190 -> [w210]
                                tunnel: [w215] -> w198
                                tunnel: w197 -> [w215]
                                tunnel: [w214] -> w192
                                tunnel: w191 -> [w214]
                                frame #0 {
                                n185 = property on="Abs. Move 2" class="DigNum (strict)"() -> ("Value"=w204:dbl)  [unwired: 2 in, 2 out]
                                n186 = call <userlib>:"Move Absolute.vi"("error in (no error)"=w203, "Position (0 units)"=w204, "Axis (1)"=w202, "VISA resource name"=w206) -> ("error out"=w201:errorcluster, "VISA resource name out"=w205:refnum<visa-resource-name>)  [unwired: 2 in]
                                }
                                frame #1 {
                                n187 = Wait (ms)(milliseconds to wait=u32 250 ("attente (ms)")) -> ()  [unwired: 1 out]
                                }
                                frame #2 {
                                n188 = Wait on Occurrence(1:TRUE ("ignorer les précédents (V)"), 2:w213) -> ()  [unwired: 1 in, 1 out]
                                }
                                frame #3 {
                                # "Tempo"
                                n189 = Wait (ms)(milliseconds to wait=u32 100 ("attente (ms)")) -> ()  [unwired: 1 out]
                                }
                                }
                                }
                                frame True {
                                }
                              }
                            }
                          }
                          n190 = Increment(x=w128) -> (x+1=w127:i32)
                          n191 = property on="Stop cycle" class="Bool (strict)"() -> ("Value"=w131:bool)  [unwired: 2 in, 2 out]
                          n192 = Greater Or Equal?(x=w127, y=w134) -> (x >= y?=w132:bool)
                          n193 = Or(x=w132, y=w131) -> (x .or. y?=w133:bool)
                        }
                      }
                      frame #2 {
                        n194 = property on="counter" class="DigNum (strict)"("Visible"=FALSE, "Value"=0 ("counter")) -> ()  [unwired: 2 in, 2 out]
                        n195 = property on="Cycle" class="Bool (strict)"("Value"=FALSE ("Cycle")) -> ()  [unwired: 2 in, 2 out]
                        n196 = property on="Stop cycle" class="Bool (strict)"("Value"=FALSE ("Cycle")) -> ()  [unwired: 2 in, 2 out]
                      }
                    }
                  }
                }
                n197 = property on="Stop polling" class="Bool (strict)"() -> ("Value"=w95:bool)  [unwired: 2 in, 2 out]
              }
              n198 = node-c288(w86) -> ()  [unwired: 1 out]
              n199 = node-c288(w84) -> ()  [unwired: 1 out]
            }
          }
        }
      }
      n200 = call <userlib>:"Close.vi"("VISA resource name"=w23) -> ()  [unwired: 10 in, 1 out]
      n201 = call <vilib>:"Simple Error Handler.vi"("error in (no error)"=w18) -> ()  [unwired: 1 in, 8 out]
      "Title" <- "ESP 301 Controller" ("Title")
    }
  }
